vi "Control-GenerateRandomSignal.vi"(2 "Parametros Maximos":T1, 3 "Sound Parameters":cluster{"# samples":u32, "tiempos (ms)":dbl}, 4 "Señal de Control IN":dbl[](array[numeric])) -> (0 "Parametros Iniciales":T1, 1 "Out":dbl[](array[numeric]))   [LabVIEW 2010]
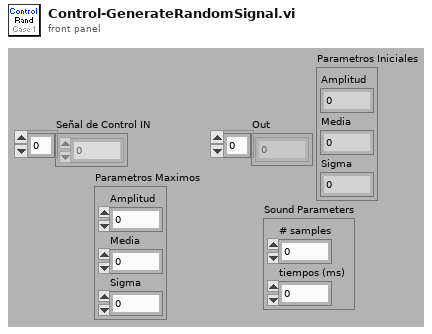
[diagram p1: front panel]
types:
  T1 = cluster{"Amplitud":dbl, "Media":dbl, "Sigma":dbl}
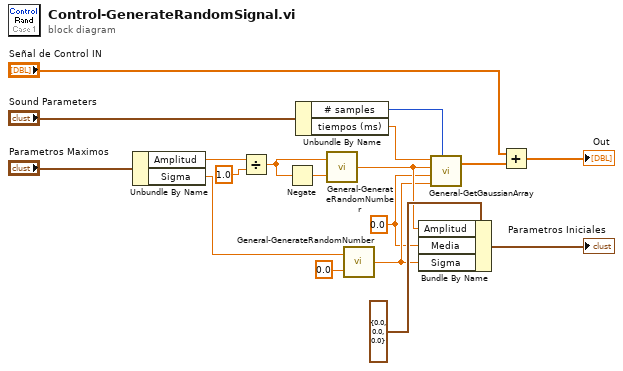
[diagram p0: block diagram]
diagram:
  w4 = 0.0 ("t0 (ms)")
  n1 = Unbundle By Name("Parametros Maximos") -> ("Amplitud"=w2:dbl, "Sigma"=w10:dbl)
  n2 = Divide(x=w2, y=1.0) -> (x/y=w3:dbl)
  n3 = Negate(x=w3) -> (-x=w14:dbl)
  n4 = Unbundle By Name("Sound Parameters") -> ("# samples"=w8:u32, "tiempos (ms)"=w7:dbl)
  n5 = call "General-GenerateRandomNumber.vi"("Min"=w14, "Max"=w3) -> ("Out"=w6:dbl)
  n6 = call "General-GenerateRandomNumber.vi"("Min"=0.0, "Max"=w10) -> ("Out"=w5:dbl)
  n7 = Bundle By Name(cluster=T1 {"Amplitud"=0.0, "Media"=0.0, "Sigma"=0.0} ("input cluster"), "Amplitud"=w6, "Media"=w4, "Sigma"=w5) -> (→"Parametros Iniciales":T1)
  n8 = call "General-GetGaussianArray.vi"("tiempo (ms)"=w7, "Amplitud"=w6, "t0 (ms)"=w4, "Sigma (ms)"=w5, "#samples"=w8) -> ("Y out"=w17:dbl[])  [unwired: 1 out]
  n9 = Add(x="Señal de Control IN", y=w17) -> (x+y=→"Out":dbl[])
